vi "Actor Core.vi"(8 "error in":errorcluster caption="错误输入", 11 "Serve in":refnum<class "Serve.lvclass"> caption="操作者输入") -> (0 "error out":errorcluster caption="错误输出", 3 "Actor out":refnum<class "Actor.lvclass"> caption="操作者输出")   [LabVIEW 2024, in "Serve.lvlib" / "Serve.lvclass"]
doc: "<p>（<strong>文件名</strong>：<span class=\"dnl\">Actor Framework.lvlib:Actor.lvclass:Actor Core.vi</span>)</p>\n<p>接收发送至操作者的消息，响应消息并处理可能导致操作者关闭的错误。</p>\n<p>子孙类重写该VI，使操作者完成特定的任务。使用<a href=\"nihelplauncher://docs/csh?context=lvcore_glang_udclass\">调用父类方法</a>节点实现重写。</p>"
uses:
  Serve.lvclass
  C:/Program Files (x86)/National Instruments/LabVIEW 2024/vi.lib/ActorFramework/Actor/Actor.lvclass
  <vilib>/ActorFramework/Actor/Actor.lvclass
  Custor/Custor/Custor.lvclass
  Serve.lvclass/Serve.ctl
  <vilib>/ActorFramework/Actor/Actor.lvclass/Actor.ctl
  <vilib>/ActorFramework/Message Enqueuer/Message Enqueuer.lvclass/Message Enqueuer.ctl
  <vilib>/ActorFramework/Message Enqueuer/Init from Existing Queue.vi
  <vilib>/ActorFramework/Message Enqueuer/Enqueue.vi
  <vilib>/ActorFramework/Stop Msg/Stop Msg.lvclass
  C:/Program Files (x86)/National Instruments/LabVIEW 2024/vi.lib/ActorFramework/Message/Message.lvclass
  <vilib>/ActorFramework/Message Priority Queue/Priority Enqueue.vi
  <vilib>/ActorFramework/Message Enqueuer/Message Enqueuer.lvclass
  <vilib>/Utility/miscctls.llb/LVStringsAndValuesArrayTypeDef_U16.ctl
panel:
  in  "下拉列表":u16(ring)
  in  "Launch":bool
  out "Log":string
  out "Receive":string
  in  "Send":bool
  in  "Msg":string
  # "Sever"
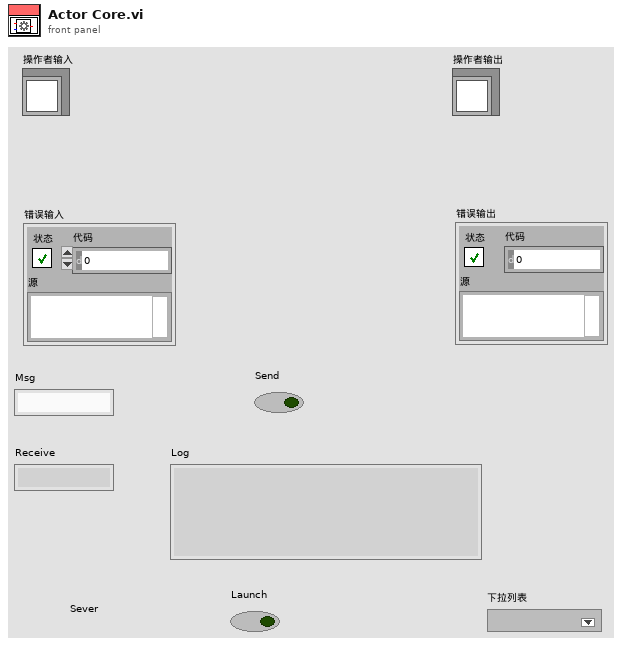
[diagram p1: front panel]
types:
  T1 = typedef "LVStringsAndValuesArrayTypeDef_U16.ctl" = cluster{"String":string, "Value":u16}[]
  T2 = enum32{"Invalid", "Standard", "Closed", "Hidden", "Minimized", "Maximized"}
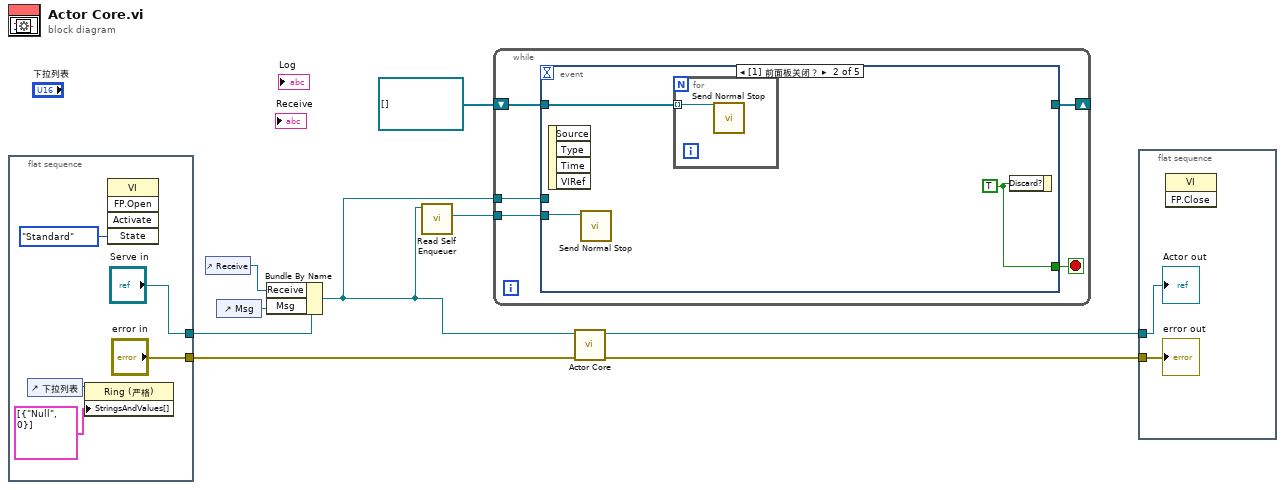
[diagram p0: block diagram]
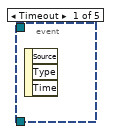
[diagram p2: hidden frame]
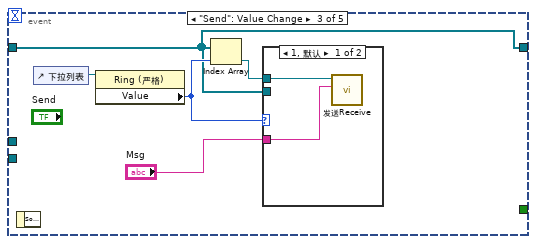
[diagram p3: hidden frame]
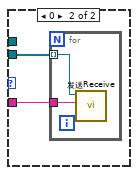
[diagram p4: hidden frame]
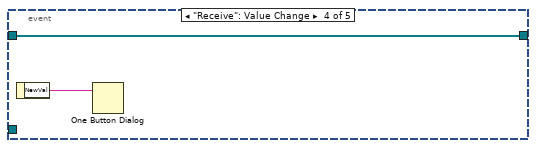
[diagram p5: hidden frame]
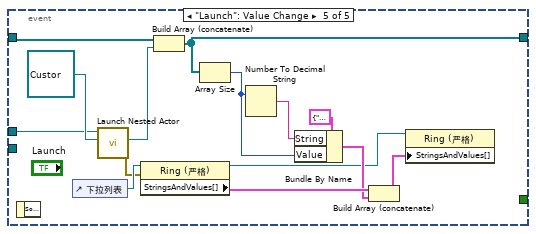
[diagram p6: hidden frame]
diagram:
  n1 = flat-sequence {
    tunnel: ["error in"] -> w4
    tunnel: ["Serve in"] -> w7
    frame #0 {
      n2 = control-ref of="下拉列表"() -> (w11:refnum<vi>)
      n3 = property class="Ring (严格)"(reference=w11, "StringsAndValues[]"=T1 [{"String"="Null", "Value"=0}] ("字符串与值[]")) -> ()  [unwired: 1 in, 2 out]
      n4 = invoke class="VI" method="FP.Open"("State"=T2."Standard" ("状态")) -> ()  [unwired: 4 in, 5 out]
    }
  }
  n5 = control-ref of="Receive"() -> (w2:refnum<vi>)
  n6 = control-ref of="Msg"() -> (w6:refnum<vi>)
  n7 = Bundle By Name(cluster=w7, "Receive"=w2, "Msg"=w6) -> (w5:refnum<class "Serve.lvclass">)
  n8 = call <vilib>:"Read Self Enqueuer.vi"("Actor"=w5) -> ("Self Enqueuer"=w3:refnum<class "Message Enqueuer.lvclass">)  [unwired: 10 in]
  n9 = while {
    tunnel: w3 -> [w19]
    tunnel: w5 -> [w17]
    shift-right: [w15] -> _
    shift-left: refnum<class "Message Enqueuer.lvclass">[] [] ("Nested Actor's Enqueuer") -> [w16]
    stop <- w18 stop-if-true
    n10 = event shown="[1] 前面板关闭？" {
      selector: _ -> [_ _ _ _ _]
      dyn-events: _ -> [_ _ _ _ _]
      timeout: _ -> [_ _ _ _ _]
      tunnel: w19 -> [_ w22 _ _ _]
      tunnel: [_ w21 _ _ _] -> w18
      tunnel: w17 -> [_ _ _ _ w49]
      tunnel: w16 -> [_ w20 w25 w35 w48]
      tunnel: [_ _ w25 w35 w44] -> w15
      event Timeout {
        n11 = event-data() -> ()  [unwired: 1 in, 3 out]
      }
      event Panel Close? {
        w21 = TRUE ("放弃？")
        n12 = event-data() -> ()  [unwired: 1 in, 4 out]
        n13 = call <vilib>:"Send Normal Stop.vi"("Message Enqueuer"=w22) -> ()  [unwired: 10 in, 1 out]
        n14 = for {
          tunnel: w20 -> [w23] mode=indexing
          n15 = call <vilib>:"Send Normal Stop.vi"("Message Enqueuer"=w23) -> ()  [unwired: 10 in, 1 out]
        }
        n16 = event-data("Discard?"=w21) -> ()  [unwired: 1 in, 1 out]
      }
      event "Send": Value Change {
        n17 = event-data() -> ()  [unwired: 1 in, 1 out]
        n18 = control-ref of="下拉列表"() -> (w28:refnum<vi>)
        n19 = property class="Ring (严格)"(reference=w28) -> ("Value"=w27:u16)  [unwired: 1 in, 2 out]
        n20 = Index Array(array=w25, index=w27) -> (element=w26:refnum<class "Message Enqueuer.lvclass">)
        n21 = case shown="1, 默认" w27 {
          tunnel: w26 -> [w30 _]
          tunnel: w25 -> [_ w31]
          tunnel: "Msg" -> [w29 w32]
          frame 1, Default {
            n22 = call "发送Receive.vi"("Receive"=w29, "Message Enqueuer"=w30) -> ()  [unwired: 8 in, 2 out]
          }
          frame 0 {
            n23 = for {
              tunnel: w32 -> [w34]
              tunnel: w31 -> [w33] mode=indexing
              n24 = call "发送Receive.vi"("Receive"=w34, "Message Enqueuer"=w33) -> ()  [unwired: 8 in, 2 out]
            }
          }
        }
      }
      event "Receive": Value Change {
        n25 = event-data() -> ("NewVal"=w36:string)  [unwired: 1 in]
        n26 = One Button Dialog(message=w36) -> ()  [unwired: 1 in, 1 out]
      }
      event "Launch": Value Change {
        n27 = event-data() -> ()  [unwired: 1 in, 1 out]
        n28 = control-ref of="下拉列表"() -> (w46:refnum<vi>)
        n29 = call <vilib>:"Launch Nested Actor.vi"("Nested Actor"=refnum<class "Custor.lvclass"> refnum ("Custor.lvlib:Custor.lvclass"), "Caller Actor in"=w49) -> ("error out"=w37:errorcluster, "Nested Actor's Enqueuer"=w47:refnum<class "Message Enqueuer.lvclass">)  [unwired: 7 in, 1 out]
        n30 = property class="Ring (严格)"(reference=w46, error in=w37) -> (reference out=w38:refnum<vi>, "StringsAndValues[]"=w45:T1)  [unwired: 1 out]
        n31 = Build Array (concatenate)(w48, w47) -> (w44:refnum<class "Message Enqueuer.lvclass">[])
        n32 = Array Size(array=w44) -> (size(s)=w41:i32)
        n33 = Number To Decimal String(number=w41) -> (decimal integer string=w42:string)  [unwired: 1 in]
        n34 = Bundle By Name(cluster=cluster{"String":string, "Value":u16} {"String"="Null", "Value"=1} ("字符串与值[]"), "String"=w42, "Value"=w41) -> (w40:cluster{"String":string, "Value":u16})
        n35 = Build Array (concatenate)(w45, w40) -> (w39:T1)
        n36 = property class="Ring (严格)"(reference=w38, "StringsAndValues[]"=w39) -> ()  [unwired: 1 in, 2 out]
      }
    }
  }
  n37 = call-parent "Actor Core.vi"("error in"=w4, "Actor in"=w5) -> ("error out"=w9:errorcluster, "Actor out"=w8:refnum<class "Actor.lvclass">)  [unwired: 8 in]
  n38 = flat-sequence {
    tunnel: w9 -> [w52]
    tunnel: w8 -> [w51]
    frame #0 {
      n39 = invoke class="VI" method="FP.Close"() -> ()  [unwired: 3 in, 3 out]
      "error out" <- w52
      "Actor out" <- w51
    }
  }
